vi "TestTimer.vi"(11 "error in (no error)":errorcluster) -> (15 "error out":errorcluster)   [LabVIEW 2016, in "TimerTest.lvlib"]
doc: "Test for Timer"
uses:
  APIs/Stimulus/VI/MakeVIFrontMost.vi
  APIs/Stimulus/ControlValue/ValueSignalLatchBooleanString.vi
  APIs/Assert/AssertControlValue/AlmostEqual.vi
  <vilib>/addons/_JKI Toolkits/Caraya/classes/Assert/Assert Almost Equal_Float.vi
  APIs/Stimulus/ControlValue/SetValueAuto.vi
  APIs/Stimulus/VI/CloseVI.vi
  TimerTest.lvlib
  <vilib>/addons/_JKI Toolkits/Caraya/classes/Test/Test.lvclass
  Drona.lvlib
  APIs/Assert/AssertControlValue/AssertControlValue.lvlib
  APIs/Stimulus/ControlValue/ControlValue.lvlib
  <vilib>/addons/_JKI Toolkits/Caraya/classes/Assert/Assert.lvclass
  APIs/Stimulus/VI/VI.lvlib
panel:
  # "TIMER TEST"
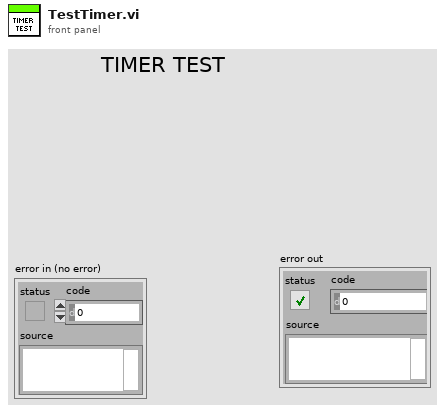
[diagram p1: front panel]
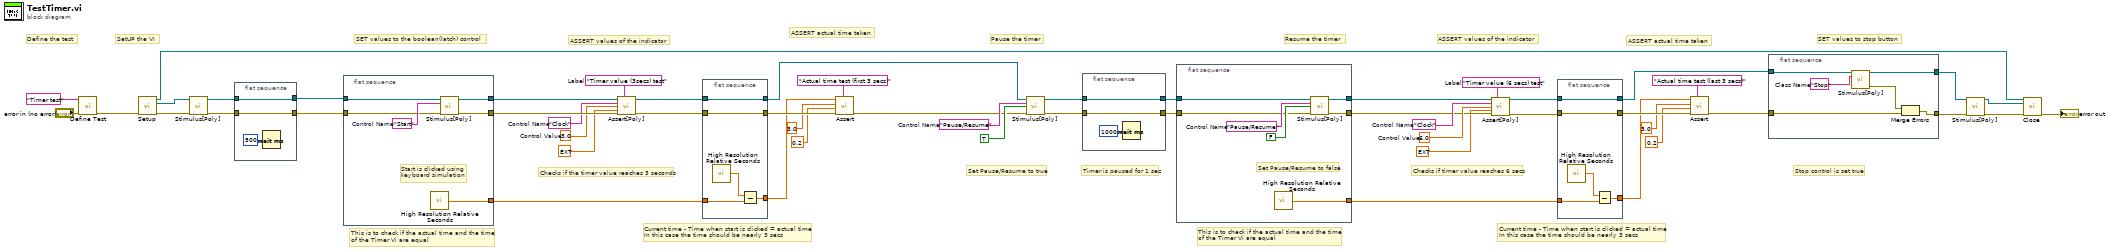
[diagram p0: block diagram]
diagram:
  w44 = "Clock"  # Control Name
  w45 = "Timer value (6 secs) test"  # Label
  w46 = 6.0  # Control Value
  w47 = "Pause/Resume"  # Control Name
  w48 = "Clock"  # Control Name
  w49 = "Timer value (3secs) test"  # Label
  w50 = 3.0  # Control Value
  # "ASSERT actual time taken"
  # "This is to check if the actual time and the time \nof the Timer Vi are equal"
  # "Current time - Time when start is clicked = actual time\nIn this case the time should be nearly 3 secs"
  # "ASSERT actual time taken"
  # "Current time - Time when start is clicked = actual time\nIn this case the time should be nearly 3 secs"
  # "This is to check if the actual time and the time \nof the Timer Vi are equal"
  # "Resume the timer"
  # "Timer is paused for 1 sec"
  # "Checks if timer value reaches 6 secs"
  # "ASSERT values of the indicator"
  # "Stop control is set true"
  # "SET values to stop button"
  # "Set Pause/Resume to true"
  # "Pause the timer"
  # "Checks if the timer value reaches 3 seconds"
  # "ASSERT values of the indicator"
  # "SET values to the boolean(latch) control"
  # "SetUP the VI"
  # "Define the test"
  n1 = call <vilib>:"Define Test.vi"("error in (no error)"="error in (no error)", "Label (VI Title)"="Timer test") -> ("error out"=w10:errorcluster)  [unwired: 9 in]
  n2 = call "Setup.vi"("error in"=w10) -> ("Application Ref"=w8:refnum<vi>, "VI Reference Out"=w7:refnum<vi>, "error out"=w6:errorcluster)  [unwired: 12 in]
  n3 = call-poly "Stimulus[Poly].vi"("VI Reference In"=w7, "error in"=w6) -> ("VI Reference Out"=w11:refnum<vi>, "error out"=w14:errorcluster)  [unwired: 12 in]
  n4 = flat-sequence {
    tunnel: w14 -> [w55]
    tunnel: [w55] -> w13
    tunnel: [w54] -> w12
    tunnel: w11 -> [w54]
    frame #0 {
      n5 = Wait (ms)(milliseconds to wait=u32 500) -> ()  [unwired: 1 out]
    }
  }
  n6 = flat-sequence {
    tunnel: [w62] -> w52
    tunnel: [w61] -> w51
    tunnel: w13 -> [w59]
    tunnel: w12 -> [w57]
    tunnel: [w58] -> w30
    frame #0 {
      w60 = "Start"  # Control Name
      # "Start is clicked using \nkeyboard simulation"
      n7 = call <vilib>:"High Resolution Relative Seconds.vi"() -> ("relative seconds"=w58:dbl)
      n8 = call-poly "Stimulus[Poly].vi"("VI Reference In"=w57, "Control Path"=w60, "error in"=w59) -> ("VI Reference Out"=w61:refnum<vi>, "error out"=w62:errorcluster)  [unwired: 11 in]
    }
  }
  n9 = call-poly "Assert[Poly].vi"("VI Reference In"=w51, "Test Label"=w49, "Control Path"=w48, "Control Value"=w50, "Tolerance"=ext 0.2, "Error In"=w52) -> ("VI Reference Out"=w32:refnum<vi>, "Error Out"=w34:errorcluster)  [unwired: 8 in]
  n10 = flat-sequence {
    tunnel: w34 -> [w67]
    tunnel: [w67] -> w33
    tunnel: w32 -> [w66]
    tunnel: [w66] -> w31
    tunnel: w30 -> [w64]
    tunnel: [w65] -> w28
    frame #0 {
      n11 = call <vilib>:"High Resolution Relative Seconds.vi"() -> ("relative seconds"=w63:dbl)
      n12 = Subtract(x=w63, y=w64) -> (x-y=w65:dbl)
    }
  }
  n13 = call-poly <vilib>:"Assert.vi"("Label"="Actual time test (first 3 secs)", "error in (no error)"=w33, "Tolerance"=0.2, "Y"=3.0, "X"=w28) -> ("error out"=w29:errorcluster)  [unwired: 6 in]
  n14 = call-poly "Stimulus[Poly].vi"("VI Reference In"=w31, "Control Path"=w47, "Value (Signaling)"=TRUE, "error in"=w29) -> ("VI Reference Out"=w40:refnum<vi>, "error out"=w41:errorcluster)  [unwired: 10 in]
  n15 = flat-sequence {
    tunnel: w41 -> [w69]
    tunnel: [w69] -> w38
    tunnel: w40 -> [w68]
    tunnel: [w68] -> w39
    frame #0 {
      n16 = Wait (ms)(milliseconds to wait=u32 1000) -> ()  [unwired: 1 out]
    }
  }
  n17 = flat-sequence {
    tunnel: w39 -> [w75]
    tunnel: w38 -> [w74]
    tunnel: [w73] -> w37
    tunnel: [w72] -> w36
    tunnel: [w71] -> w18
    frame #0 {
      w76 = "Pause/Resume"  # Control Name
      # "Set Pause/Resume to false"
      n18 = call <vilib>:"High Resolution Relative Seconds.vi"() -> ("relative seconds"=w71:dbl)
      n19 = call-poly "Stimulus[Poly].vi"("VI Reference In"=w75, "Control Path"=w76, "Value (Signaling)"=FALSE, "error in"=w74) -> ("VI Reference Out"=w72:refnum<vi>, "error out"=w73:errorcluster)  [unwired: 10 in]
    }
  }
  n20 = call-poly "Assert[Poly].vi"("VI Reference In"=w36, "Test Label"=w45, "Control Path"=w44, "Control Value"=w46, "Tolerance"=ext 0.2, "Error In"=w37) -> ("VI Reference Out"=w17:refnum<vi>, "Error Out"=w19:errorcluster)  [unwired: 8 in]
  n21 = flat-sequence {
    tunnel: w19 -> [w82]
    tunnel: [w82] -> w24
    tunnel: w17 -> [w81]
    tunnel: [w81] -> w16
    tunnel: w18 -> [w79]
    tunnel: [w80] -> w23
    frame #0 {
      n22 = call <vilib>:"High Resolution Relative Seconds.vi"() -> ("relative seconds"=w78:dbl)
      n23 = Subtract(x=w78, y=w79) -> (x-y=w80:dbl)
    }
  }
  n24 = call-poly <vilib>:"Assert.vi"("Label"="Actual time test (last 3 secs)", "error in (no error)"=w24, "Tolerance"=0.2, "Y"=3.0, "X"=w23) -> ("error out"=w15:errorcluster)  [unwired: 6 in]
  n25 = flat-sequence {
    tunnel: [w86] -> w4
    tunnel: [w87] -> w2
    tunnel: w16 -> [w85]
    tunnel: w15 -> [w83]
    frame #0 {
      w88 = "Stop"  # Class Name
      n26 = call-poly "Stimulus[Poly].vi"("VI Reference In"=w85, "Control Path"=w88) -> ("VI Reference Out"=w87:refnum<vi>, "error out"=w84:errorcluster)  [unwired: 12 in]
      n27 = Merge Errors(w84, w83) -> (w86:errorcluster)
    }
  }
  n28 = call-poly "Stimulus[Poly].vi"("VI Reference In"=w2, "error in"=w4) -> ("VI Reference Out"=w1:refnum<vi>, "error out"=w3:errorcluster)  [unwired: 12 in]
  n29 = call "Close.vi"("Application Ref"=w8, "VI Reference"=w1, "error in"=w3) -> ("error out"=→"error out":errorcluster)  [unwired: 12 in]
